vi "Initialize.vi"(8 "error in (no error)":errorcluster, 9 "Reset (True)":bool=TRUE, 10 "ID Query (True)":bool=TRUE, 11 "VISA resource name":refnum<visa-resource-name>) -> (0 "error out":errorcluster, 3 "VISA resource name out":refnum<visa-resource-name>)   [LabVIEW 2021, in "Yokogawa WT1800 Series.lvlib"]
doc: "Establishes communication with the instrument and optionally performs an instrument identification query and/or an instrument reset. It also places the instrument in a default state needed for other instrument driver operations. Therefore, call this VI before calling other instrument driver VIs for this instrument. Generally, you need to call the <B>Initialize VI</B> only once at the beginning of an application."
uses:
  <instrlib>/Yokogawa WT1800 Series/Yokogawa WT1800 Series.lvlib
panel:
  # "(c) 2011 Yokogawa Meters & Instruments.  All rights reserved."
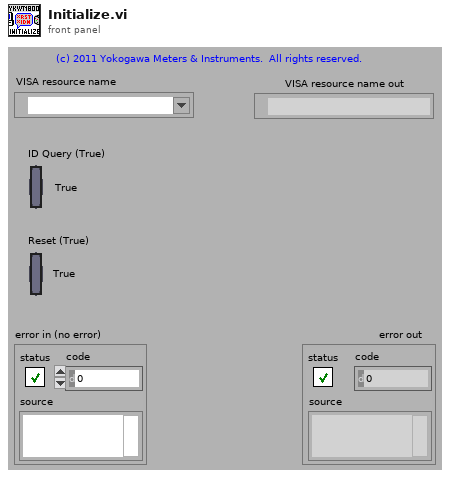
[diagram p1: front panel]
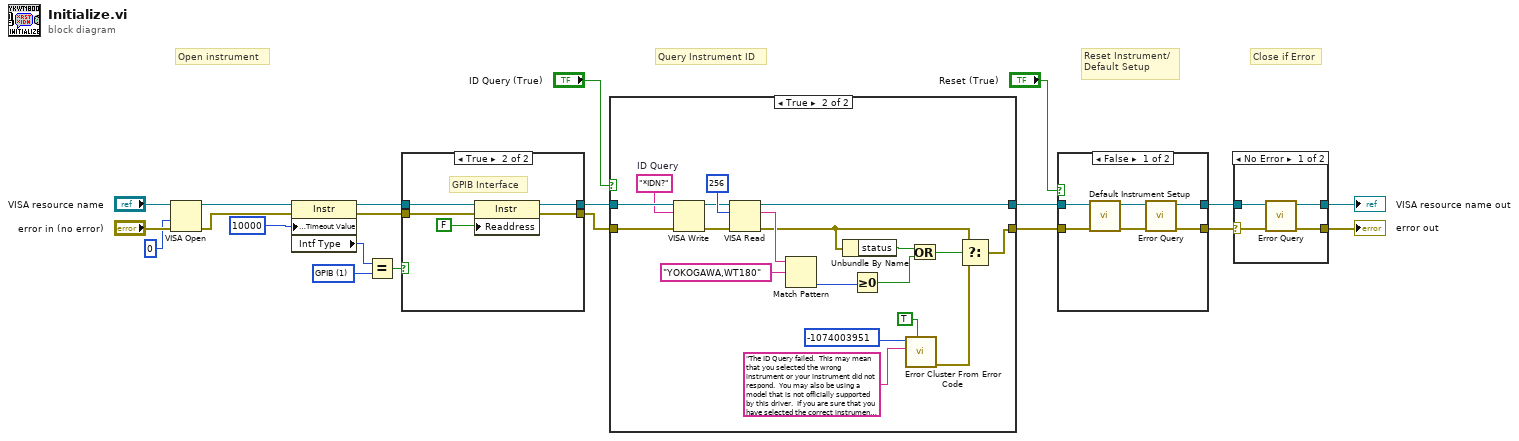
[diagram p0: block diagram]
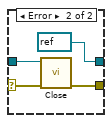
[diagram p3: hidden frame]
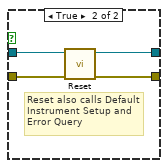
[diagram p4: hidden frame]
diagram:
  w7 = u16 1 items=["GPIB"=1, "VXI"=2, "GPIB-VXI"=3, "Serial"=4, "PXI"=5, "TCPIP"=6, "USB"=7, "FireWire"=9] ("Interface Information:Interface Type")
  # "Close if Error"
  # "Query Instrument ID"
  # "Reset Instrument/\nDefault Setup"
  # "Open instrument"
  n1 = VISA Open(access mode=u32 0, error in (no error)="error in (no error)", VISA resource name="VISA resource name") -> (VISA resource name=w10:refnum<visa-resource-name>, error out=w9:errorcluster)  [unwired: 2 in]
  n2 = property class="Instr"(reference=w10, error in=w9, "General Settings:Timeout Value"=u32 10000) -> (reference out=w4:refnum<visa-resource-name>, error out=w2:errorcluster, "Intf Type"=w6:u16)
  n3 = Equal?(x=w6, y=w7) -> (x = y?=w5:bool)
  n4 = case shown="True" w5 {
    tunnel: w4 -> [w23 w27]
    tunnel: [w23 w26] -> w3
    tunnel: w2 -> [w22 w25]
    tunnel: [w22 w24] -> w1
    frame False {
      # "TCP/IP, and USB Interface"
    }
    frame True {
      # "GPIB Interface"
      n5 = property class="Instr"(reference=w27, error in=w25, "Readdress"=FALSE ("GPIB Settings:Readdressing")) -> (reference out=w26:refnum<visa-resource-name>, error out=w24:errorcluster)
    }
  }
  n6 = case shown="True" "ID Query (True)" {
    tunnel: [w29 w49] -> w20
    tunnel: [w30 w46] -> w21
    tunnel: w3 -> [w30 w47]
    tunnel: w1 -> [w29 w48]
    frame False {
    }
    frame True {
      w42 = "*IDN?"  # ID Query
      n7 = VISA Write(VISA resource name=w47, write buffer=w42, error in (no error)=w48) -> (VISA resource name out=w32:refnum<visa-resource-name>, error out=w31:errorcluster)  [unwired: 1 out]
      n8 = VISA Read(VISA resource name=w32, byte count=u32 256, error in (no error)=w31) -> (VISA resource name out=w46:refnum<visa-resource-name>, read buffer=w45:string, error out=w36:errorcluster)  [unwired: 1 out]
      n9 = Match Pattern(string=w45, regular expression="YOKOGAWA,WT180") -> (offset past match=w37:i32)  [unwired: 1 in, 3 out]
      n10 = Unbundle By Name(w36) -> ("status"=w35:bool)
      n11 = Greater Or Equal To 0?(x=w37) -> (x >= 0?=w33:bool)
      n12 = call <vilib>:"Error Cluster From Error Code.vi"("show call chain? (False)"=TRUE, "error message (\"\")"="The ID Query failed.  This may mean that you selected the wrong instrument or your instrument did not respond.  You may also be using a model that is not officially supported by this driver.  If you are sure that you have selected the correct instrument and it is responding, try disabling the ID Query." ("Source (VI Name)"), "error code (0)"=-1074003951 ("Code")) -> ("error out"=w41:errorcluster)  [unwired: 6 in]
      n13 = Or(x=w35, y=w33) -> (x .or. y?=w34:bool)
      n14 = Select(t=w36, s=w34, f=w41) -> (s? t:f=w49:errorcluster)
    }
  }
  n15 = case shown="False" "Reset (True)" {
    tunnel: w20 -> [w54 w56]
    tunnel: [w50 w59] -> w13
    tunnel: w21 -> [w55 w57]
    tunnel: [w52 w58] -> w14
    frame False {
      n16 = call <instrlib>:"Default Instrument Setup.vi"("error in (no error)"=w54, "VISA resource name"=w55) -> ("error out"=w51:errorcluster, "VISA resource name out"=w53:refnum<visa-resource-name>)  [unwired: 8 in]
      n17 = call <instrlib>:"Error Query.vi"("error in (no error)"=w51, "VISA resource name"=w53) -> ("error out"=w50:errorcluster, "VISA resource name out"=w52:refnum<visa-resource-name>)  [unwired: 6 in, 2 out]
    }
    frame True {
      # "Reset also calls Default Instrument Setup and Error Query"
      n18 = call <instrlib>:"Reset.vi"("error in (no error)"=w56, "VISA resource name"=w57) -> ("error out"=w59:errorcluster, "VISA resource name out"=w58:refnum<visa-resource-name>)  [unwired: 8 in]
    }
  }
  n19 = case shown="No Error" w13 {
    selector: w13 -> [w61 w65]
    tunnel: w14 -> [w60 w66]
    tunnel: [w63 refnum<visa-resource-name> refnum ("VISA resource name out")] -> w12
    tunnel: [w62 w67] -> w11
    frame No Error {
      n20 = call <instrlib>:"Error Query.vi"("error in (no error)"=w61, "VISA resource name"=w60) -> ("error out"=w62:errorcluster, "VISA resource name out"=w63:refnum<visa-resource-name>)  [unwired: 6 in, 2 out]
    }
    frame Error {
      n21 = call <instrlib>:"Close.vi"("error in (no error)"=w65, "VISA resource name"=w66) -> ("error out"=w67:errorcluster)  [unwired: 9 in]
    }
  }
  "VISA resource name out" <- w12
  "error out" <- w11
